vi "USBCamera.vi"() -> ()   [LabVIEW 2012]
uses:
  <vilib>/userdefined/High Color/IMAQdx.ctl
  <vilib>/vision/driver/NI_Vision_Acquisition_Software.lvlib
panel:
  in  "Tab Control":enum32{"Camera", "Cursors", "C & M"}(tab)
  in  "Close":bool
  in  "Open":bool
  in  "Session In":T1
  in  "Avi Path":path
  in  "Stop":bool
  in  "Record":bool
  in  "Slide":dbl(slide) scale=-240.0..240.0
  in  "Cursor.Visible":bool
  in  "Slide 2":dbl(slide) scale=-240.0..240.0
  in  "Cursor.Visible 2":bool
  in  "Slide 3":dbl(slide) scale=-240.0..240.0
  in  "Cursor.Visible 3":bool
  in  "Slide 4":dbl(slide) scale=-240.0..240.0
  in  "Cursor.Visible 4":bool
  in  "Slide 5":dbl(slide) scale=-240.0..240.0
  in  "Cursor.Visible 5":bool
  in  "Set":bool
  in  "M":dbl
  out "D3":dbl
  in  "D2":dbl
  in  "D1":dbl
  out "N3":dbl
  in  "N2":dbl
  in  "N1":dbl
  in  "Calculate":bool
  out "Result":dbl
  out "C3":dbl
  in  "C2":dbl
  in  "C1":dbl
  out "Waveform Graph":dbl[](graph)
  out "Image":T2(plugin-control)
  # "USB 摄像头控制程序"
  # "Cam"
  # "Cursor 1"
  # "Cursor 2"
  # "Cursor 3"
  # "Cursor 4"
  # "Cursor 5"
  # "Cursor / pixel"
  # "Distance / mm"
  # "Cursor / pixel"
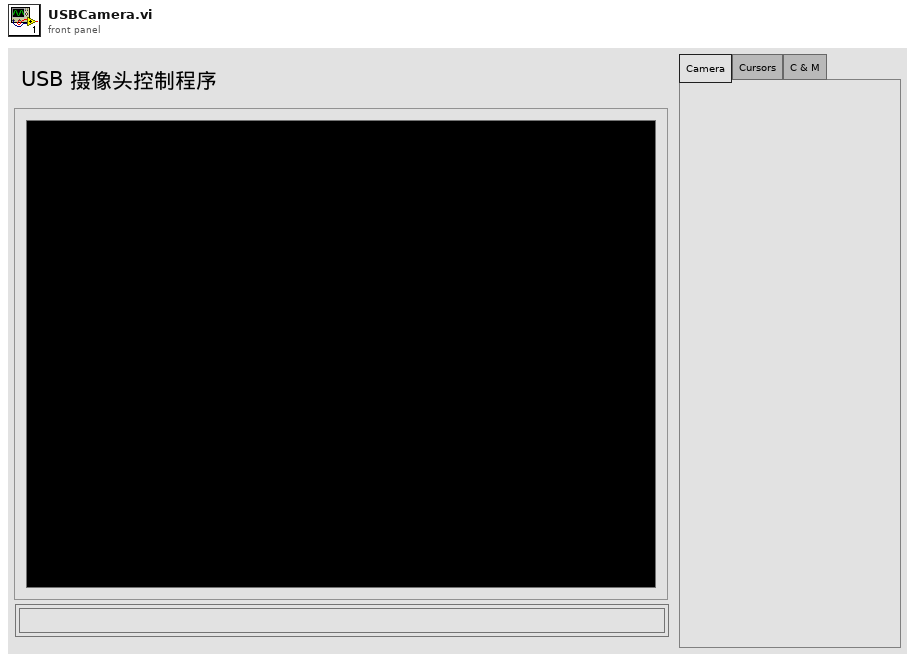
[diagram p1: front panel]
types:
  T1 = typedef "IMAQdx.ctl" = refnum<k21>
  T2 = typedef "IMAQ Image.ctl" = refnum<image>
  T3 = enum8{"Enabled", "Disabled", "Disabled and Grayed Out"}
  T4 = typedef "Image Type" = u32
  T5 = typedef "AviRefnum.ctl" = refnum<k1>
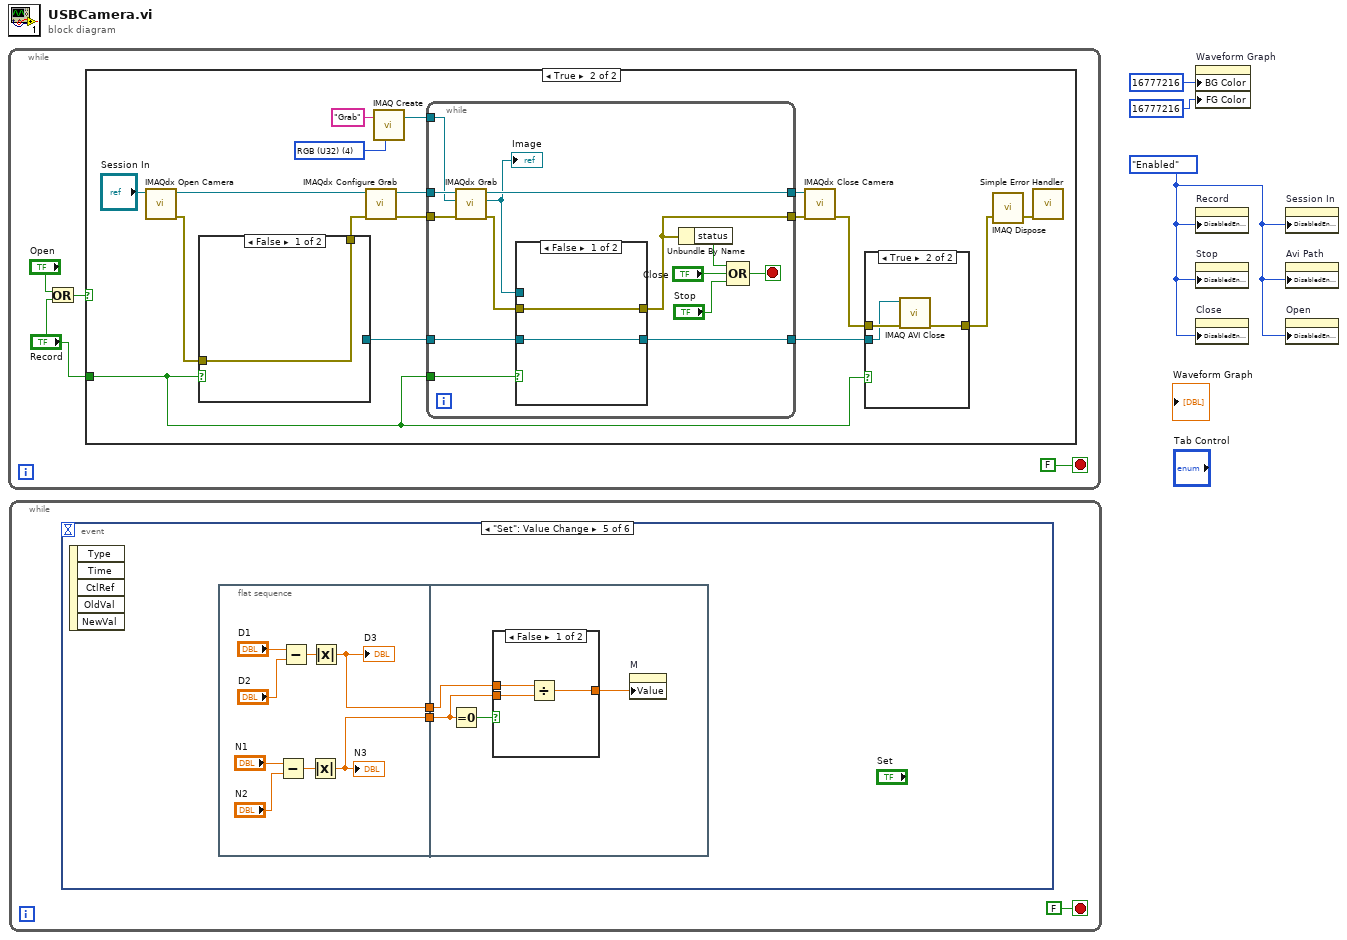
[diagram p0: block diagram]
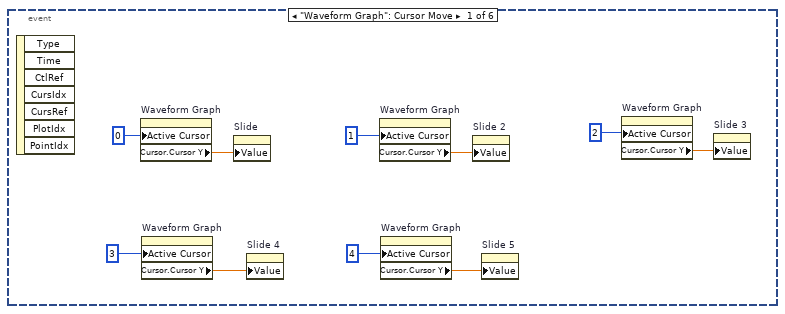
[diagram p2: hidden frame]
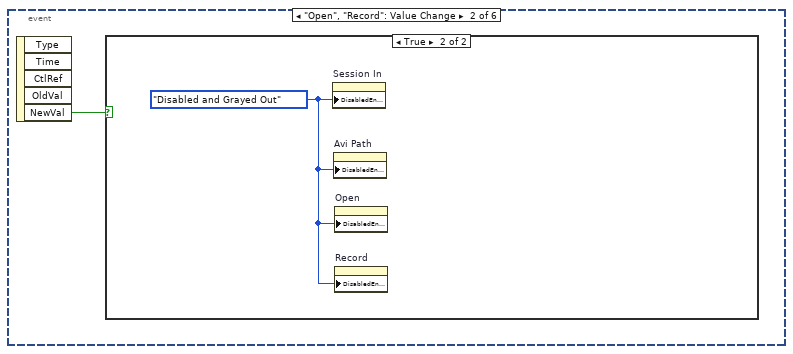
[diagram p3: hidden frame]
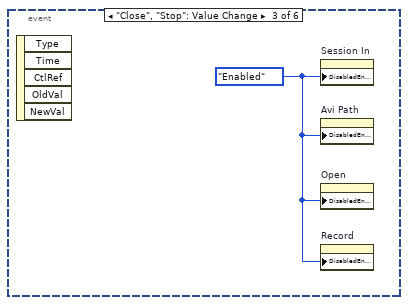
[diagram p5: hidden frame]
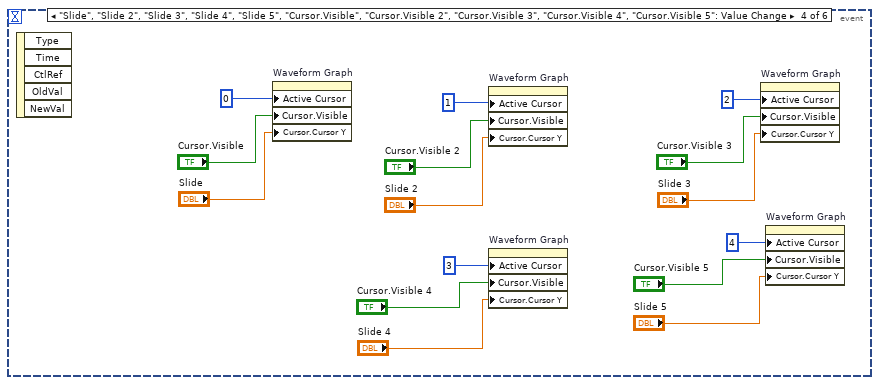
[diagram p6: hidden frame]
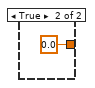
[diagram p7: hidden frame]
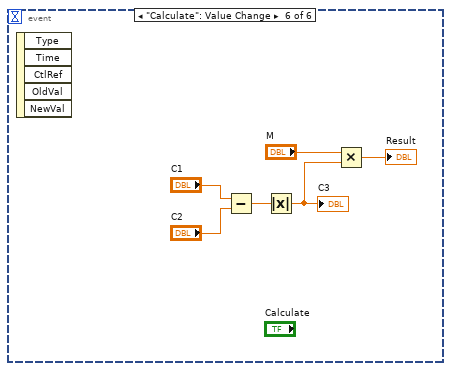
[diagram p8: hidden frame]
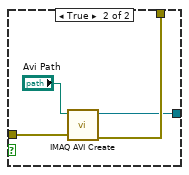
[diagram p11: hidden frame]
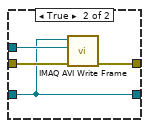
[diagram p12: hidden frame]
diagram:
  w1 = T3."Enabled" ("Disabled")
  n1 = while {
    stop <- FALSE stop-if-true
    n2 = Or(x="Open", y="Record") -> (x .or. y?=w6:bool)
    n3 = case shown="True" w6 {
      tunnel: "Record" -> [_ w11]
      frame False {
      }
      frame True {
        w21 = T4 4 items=["Grayscale (U8)", "Grayscale (I16)", "Grayscale (SGL)", "Complex (CSG)", "RGB (U32)", "HSL (U32)", "RGB (U64)", "Grayscale (U16)"] ("Image Type")
        n4 = call <vilib>:"IMAQdx Open Camera.vi"("Session In"="Session In") -> ("error out"=w15:errorcluster, "Session Out"=w13:T1)  [unwired: 9 in]
        n5 = case shown="False" w11 {
          tunnel: w15 -> [w29 w33]
          tunnel: [w29 w32] -> w14
          tunnel: [_ w31] -> w12
          frame False {
          }
          frame True {
            n6 = call "IMAQ AVI Create"("error in (no error)"=w33, "AVI Path"="Avi Path") -> ("error out"=w32:errorcluster, "Avi Refnum"=w31:T5)  [unwired: 8 in]
          }
        }
        n7 = call <vilib>:"IMAQdx Configure Grab.vi"("error in"=w14, "Session In"=w13) -> ("error out"=w16:errorcluster, "Session Out"=w17:T1)  [unwired: 8 in]
        n8 = call "IMAQ Create"("Image Name"="Grab", "Image Type"=w21) -> ("New Image"=w23:T2)  [unwired: 3 in, 1 out]
        n9 = while {
          tunnel: w17 -> [w47]
          tunnel: w16 -> [w46]
          tunnel: w23 -> [w45]
          tunnel: [w44] -> w20
          tunnel: [w38] -> w19
          tunnel: w12 -> [w42]
          tunnel: w11 -> [w40]
          tunnel: [w39] -> w8
          stop <- w34 stop-if-true
          n10 = call <vilib>:"IMAQdx Grab.vi"("error in"=w46, "Image In"=w45, "Session In"=w47) -> ("error out"=w41:errorcluster, "Image Out"=w43:T2, "Session Out"=w44:T1)  [unwired: 5 in, 1 out]
          "Image" <- w43
          n11 = case shown="False" w40 {
            tunnel: w43 -> [_ w53]
            tunnel: w42 -> [w48 w50]
            tunnel: w41 -> [w49 w52]
            tunnel: [w49 w51] -> w38
            tunnel: [w48 w50] -> w39
            frame False {
            }
            frame True {
              n12 = call "IMAQ AVI Write Frame"("error in (no error)"=w52, "Image"=w53, "Avi Refnum"=w50) -> ("error out"=w51:errorcluster)  [unwired: 7 in, 1 out]
            }
          }
          n13 = Unbundle By Name(w38) -> ("status"=w37:bool)
          n14 = Compound Arithmetic op=OR(w37, "Close", "Stop") -> (w34:bool)
        }
        n15 = call <vilib>:"IMAQdx Close Camera.vi"("error in"=w19, "Session In"=w20) -> ("error out"=w10:errorcluster)  [unwired: 9 in]
        n16 = case shown="True" w11 {
          tunnel: w10 -> [w25 w27]
          tunnel: [w25 w28] -> w9
          tunnel: w8 -> [_ w26]
          frame False {
          }
          frame True {
            n17 = call "IMAQ AVI Close"("error in (no error)"=w27, "Avi Refnum"=w26) -> ("error out"=w28:errorcluster)  [unwired: 9 in]
          }
        }
        n18 = call "IMAQ Dispose"("error in (no error)"=w9) -> ("error out"=w18:errorcluster)  [unwired: 5 in]
        n19 = call <vilib>:"Simple Error Handler.vi"("error in (no error)"=w18) -> ()  [unwired: 4 in, 5 out]
      }
    }
  }
  n20 = while {
    stop <- FALSE stop-if-true
    n21 = event shown="[4] \"Set\": Value Change" {
      selector: _ -> [_ _ _ _ _ _]
      dyn-events: _ -> [_ _ _ _ _ _]
      timeout: _ -> [_ _ _ _ _ _]
      event "Waveform Graph": Cursor Move {
        n22 = event-data() -> ()  [unwired: 1 in, 7 out]
        n23 = property on="Waveform Graph" class="WFGraph (strict)"("Active Cursor"=u32 0) -> ("Cursor.Cursor Y"=w61:dbl)  [unwired: 2 in, 2 out]
        n24 = property on="Waveform Graph" class="WFGraph (strict)"("Active Cursor"=u32 3) -> ("Cursor.Cursor Y"=w56:dbl)  [unwired: 2 in, 2 out]
        n25 = property on="Slide" class="Slide (strict)"("Value"=w61) -> ()  [unwired: 2 in, 2 out]
        n26 = property on="Slide 4" class="Slide (strict)"("Value"=w56) -> ()  [unwired: 2 in, 2 out]
        n27 = property on="Waveform Graph" class="WFGraph (strict)"("Active Cursor"=u32 1) -> ("Cursor.Cursor Y"=w60:dbl)  [unwired: 2 in, 2 out]
        n28 = property on="Waveform Graph" class="WFGraph (strict)"("Active Cursor"=u32 4) -> ("Cursor.Cursor Y"=w55:dbl)  [unwired: 2 in, 2 out]
        n29 = property on="Slide 2" class="Slide (strict)"("Value"=w60) -> ()  [unwired: 2 in, 2 out]
        n30 = property on="Slide 5" class="Slide (strict)"("Value"=w55) -> ()  [unwired: 2 in, 2 out]
        n31 = property on="Waveform Graph" class="WFGraph (strict)"("Active Cursor"=u32 2) -> ("Cursor.Cursor Y"=w59:dbl)  [unwired: 2 in, 2 out]
        n32 = property on="Slide 3" class="Slide (strict)"("Value"=w59) -> ()  [unwired: 2 in, 2 out]
      }
      event "Open", "Record": Value Change {
        n33 = event-data() -> ("NewVal"=w65:bool)  [unwired: 1 in, 4 out]
        n34 = case shown="True" w65 {
          frame False {
          }
          frame True {
            w66 = T3."Disabled and Grayed Out" ("Disabled")
            n35 = property on="Session In" class="IMAQdx (strict)"("DisabledEnum"=w66) -> ()  [unwired: 2 in, 2 out]
            n36 = property on="Avi Path" class="Path"("DisabledEnum"=w66) -> ()  [unwired: 2 in, 2 out]
            n37 = property on="Open" class="Bool"("DisabledEnum"=w66) -> ()  [unwired: 2 in, 2 out]
            n38 = property on="Record" class="Bool"("DisabledEnum"=w66) -> ()  [unwired: 2 in, 2 out]
          }
        }
      }
      event "Close", "Stop": Value Change {
        w67 = T3."Enabled" ("Disabled")
        n39 = event-data() -> ()  [unwired: 1 in, 5 out]
        n40 = property on="Session In" class="IMAQdx (strict)"("DisabledEnum"=w67) -> ()  [unwired: 2 in, 2 out]
        n41 = property on="Avi Path" class="Path"("DisabledEnum"=w67) -> ()  [unwired: 2 in, 2 out]
        n42 = property on="Open" class="Bool"("DisabledEnum"=w67) -> ()  [unwired: 2 in, 2 out]
        n43 = property on="Record" class="Bool"("DisabledEnum"=w67) -> ()  [unwired: 2 in, 2 out]
      }
      event "Slide", "Slide 2", "Slide 3", "Slide 4", "Slide 5", "Cursor.Visible", "Cursor.Visible 2", "Cursor.Visible 3", "Cursor.Visible 4", "Cursor.Visible 5": Value Change {
        n44 = event-data() -> ()  [unwired: 1 in, 5 out]
        n45 = property on="Waveform Graph" class="WFGraph (strict)"("Active Cursor"=u32 0, "Cursor.Visible"="Cursor.Visible", "Cursor.Cursor Y"="Slide") -> ()  [unwired: 2 in, 2 out]
        n46 = property on="Waveform Graph" class="WFGraph (strict)"("Active Cursor"=u32 1, "Cursor.Visible"="Cursor.Visible 2", "Cursor.Cursor Y"="Slide 2") -> ()  [unwired: 2 in, 2 out]
        n47 = property on="Waveform Graph" class="WFGraph (strict)"("Active Cursor"=u32 3, "Cursor.Visible"="Cursor.Visible 4", "Cursor.Cursor Y"="Slide 4") -> ()  [unwired: 2 in, 2 out]
        n48 = property on="Waveform Graph" class="WFGraph (strict)"("Active Cursor"=u32 2, "Cursor.Visible"="Cursor.Visible 3", "Cursor.Cursor Y"="Slide 3") -> ()  [unwired: 2 in, 2 out]
        n49 = property on="Waveform Graph" class="WFGraph (strict)"("Active Cursor"=u32 4, "Cursor.Visible"="Cursor.Visible 5", "Cursor.Cursor Y"="Slide 5") -> ()  [unwired: 2 in, 2 out]
      }
      event "Set": Value Change {
        n50 = event-data() -> ()  [unwired: 1 in, 5 out]
        n51 = flat-sequence {
          tunnel: [w86] -> w84
          tunnel: [w85] -> w83
          tunnel: w84 -> [w95]
          tunnel: w83 -> [w94]
          frame #0 {
            n52 = Subtract(x="N1", y="N2") -> (x-y=w90:dbl)
            n53 = Subtract(x="D1", y="D2") -> (x-y=w87:dbl)
            n54 = Absolute Value(x=w90) -> (abs(x)=w85:dbl)
            "N3" <- w85
            n55 = Absolute Value(x=w87) -> (abs(x)=w86:dbl)
            "D3" <- w86
          }
          frame #1 {
            n56 = Equal To 0?(x=w94) -> (x = 0?=w96:bool)
            n57 = case shown="False" w96 {
              tunnel: w95 -> [w99 _]
              tunnel: w94 -> [w98 _]
              tunnel: [w97 0.0] -> w93
              frame False {
                n58 = Divide(x=w99, y=w98) -> (x/y=w97:dbl)
              }
              frame True {
              }
            }
            n59 = property on="M" class="DigNum (strict)"("Value"=w93) -> ()  [unwired: 2 in, 2 out]
          }
        }
      }
      event "Calculate": Value Change {
        n60 = event-data() -> ()  [unwired: 1 in, 5 out]
        n61 = Subtract(x="C1", y="C2") -> (x-y=w106:dbl)
        n62 = Absolute Value(x=w106) -> (abs(x)=w103:dbl)
        "C3" <- w103
        n63 = Multiply(x="M", y=w103) -> (x*y=→"Result":dbl)
      }
    }
  }
  n64 = property on="Waveform Graph" class="WFGraph (strict)"("BG Color"=u32 16777216 ("Plot Area:Colors:BG Color"), "FG Color"=u32 16777216 ("Plot Area:Colors:FG Color")) -> ()  [unwired: 2 in, 2 out]
  n65 = property on="Record" class="Bool"("DisabledEnum"=w1) -> ()  [unwired: 2 in, 2 out]
  n66 = property on="Stop" class="Bool"("DisabledEnum"=w1) -> ()  [unwired: 2 in, 2 out]
  n67 = property on="Close" class="Bool"("DisabledEnum"=w1) -> ()  [unwired: 2 in, 2 out]
  n68 = property on="Session In" class="IMAQdx (strict)"("DisabledEnum"=w1) -> ()  [unwired: 2 in, 2 out]
  n69 = property on="Avi Path" class="Path"("DisabledEnum"=w1) -> ()  [unwired: 2 in, 2 out]
  n70 = property on="Open" class="Bool"("DisabledEnum"=w1) -> ()  [unwired: 2 in, 2 out]
